vi "Parse Data JSON.vi"(8 "error in (no error)":errorcluster, 10 "JSON String":string, 11 "Event in":refnum<class "Event.lvclass">) -> (0 "error out":errorcluster, 1 "Typed?":bool, 2 "Typed Message":refnum<class "Response.lvclass">, 3 "Event out":refnum<class "Event.lvclass">)   [LabVIEW 2022 SP3, in "obs-websocket-lv.lvlib" / "Event.lvclass"]
uses:
  Event.lvclass
  Event.lvclass/Event.ctl
  <vilib>/IlluminatedG/lv-web-crypto/lv-json/JSON/JSON.lvlib
  Response/Response.lvclass
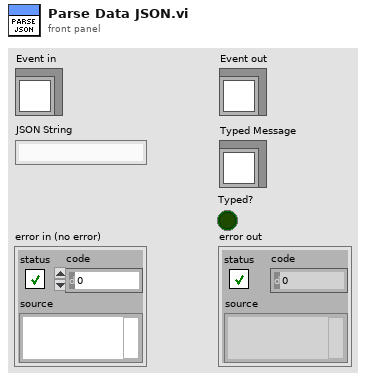
[diagram p1: front panel]
types:
  T1 = typedef "JSON.lvlib/JSON Item Type.ctl" = enum16{"unknown", "null", "Array", "Object", "String", "Number", "Boolean"}
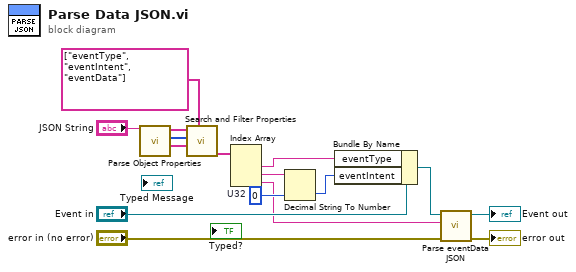
[diagram p0: block diagram]
diagram:
  w8 = u32 0  # U32
  n1 = call <vilib>:"Parse Object Properties.vi"("JSON String"="JSON String") -> ("Values"=w12:string[], "Item Types"=w13:T1[], "Keys"=w14:string[])  [unwired: 7 in, 1 out]
  n2 = call <vilib>:"Search and Filter Properties.vi"("Search Keys"=string[] ["eventType", "eventIntent", "eventData"], "Values In"=w12, "Types In"=w13, "Keys In"=w14) -> ("Filtered Values"=w10:string[])  [unwired: 2 in, 5 out]
  n3 = Index Array(array=w10) -> (element #1=w7:string, element #2=w9:string, element #3=w3:string)  [unwired: 3 in]
  n4 = Decimal String To Number(string=w9, default (0L)=w8) -> (number=w6:u32)  [unwired: 1 in, 1 out]
  n5 = Bundle By Name(cluster="Event in", "eventType"=w7, "eventIntent"=w6) -> (w4:refnum<class "Event.lvclass">)
  n6 = call-dynamic "Parse eventData JSON.vi"("error in (no error)"="error in (no error)", "eventData JSON"=w3, "Event in"=w4) -> ("error out"=→"error out":errorcluster, "Event out"=→"Event out":refnum<class "Event.lvclass">)  [unwired: 7 in]
